vi "Initialize.vi"(8 "error in":errorcluster, 9 "Number of Channels":u32=1, 10 "Plugin Name":string, 11 "Voltage Limits in":refnum<class "Voltage Limits.lvclass">) -> (0 "error out":errorcluster, 3 "Voltage Limits out":refnum<class "Voltage Limits.lvclass">)   [LabVIEW 2023, in "Voltage Limits.lvclass"]
uses:
  Voltage Limits.lvclass
  Voltage Limits.lvclass/Voltage Limits.ctl
  <vilib>/ADAS Replay HIL/Channels/Tag Wrapper/Polymorphic/Open Consumer Tag (Double).vi
  <vilib>/ADAS Replay HIL/Channels/Tag Wrapper/Polymorphic/Set Default Value (Double).vi
  <vilib>/ADAS Replay HIL/Channels/Tag Wrapper/Polymorphic/Open Consumer Tag (Double).vi/bacb721e-673a-491a-accd-959f2e1f334e.vi
  <vilib>/ADAS Replay HIL/Channels/Tag Wrapper/Polymorphic/Set Default Value (Double).vi/228e99de-6fcf-414d-86fc-dc277c7b351f.vi
  <vilib>/ADAS Replay HIL/Channels/Tag Wrapper/Polymorphic/Open Consumer Tag (Double).vi/bacb721e-673a-491a-accd-959f2e1f334e.vi/c28b0ead-42ad-4072-80a2-aca7f2bd7ce3.vi
  <vilib>/ADAS Replay HIL/Channels/Tag Wrapper/Polymorphic/Set Default Value (Double).vi/228e99de-6fcf-414d-86fc-dc277c7b351f.vi/4bc1c15b-36ab-481f-b8dd-c64075ce723a.vi
  <vilib>/ADAS Replay HIL/AdasHilServices/AdasHilServices Fill In Error Info Ex.vi
  <vilib>/ADAS Replay HIL/Channels/Tag Wrapper/Tag Wrapper.lvlib
  Capability/Capability.lvclass
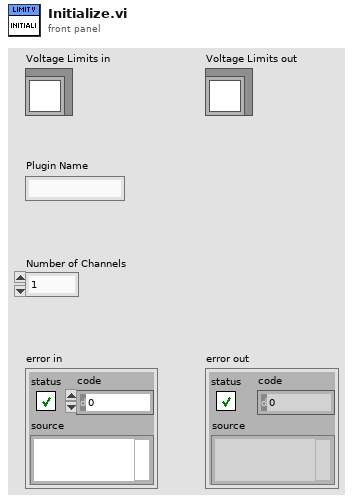
[diagram p1: front panel]
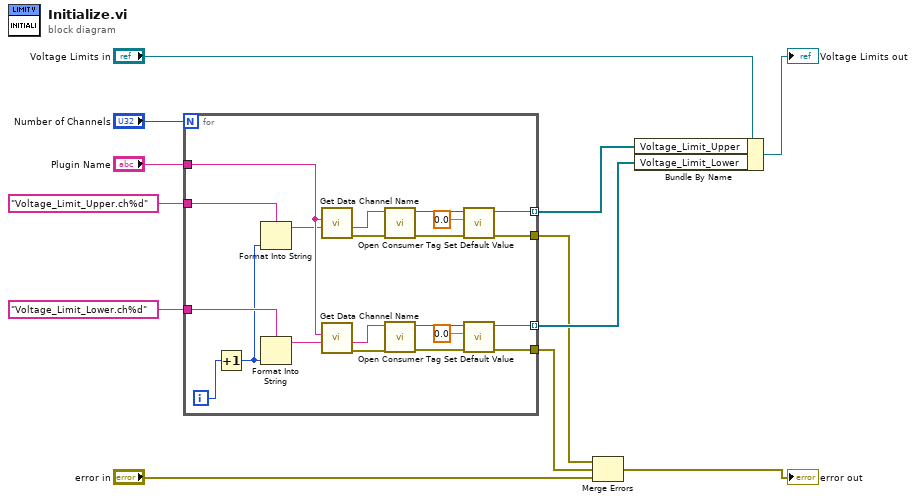
[diagram p0: block diagram]
diagram:
  n1 = for {
    N: "Number of Channels" -> [_]
    tunnel: [w29] -> w10 mode=indexing
    tunnel: [w28] -> w9 mode=indexing
    tunnel: [w27] -> w8
    tunnel: [w26] -> w7
    tunnel: "Plugin Name" -> [w25]
    tunnel: "Voltage_Limit_Upper.ch%d" ("Channel Name") -> [w17]
    tunnel: "Voltage_Limit_Lower.ch%d" ("Channel Name") -> [w15]
    i -> [w14]
    n2 = Increment(x=w14) -> (x+1=w13:i32)
    n3 = Format Into String(format string=w17, w13) -> (resulting string=w18:string)  [unwired: 2 in, 1 out]
    n4 = Format Into String(format string=w15, w13) -> (resulting string=w16:string)  [unwired: 2 in, 1 out]
    n5 = call "Get Data Channel Name.vi"("Channel Name"=w18, "Plugin Name"=w25) -> ("error out"=w22:errorcluster, "Data Channel Name"=w21:string)  [unwired: 8 in]
    n6 = call "Get Data Channel Name.vi"("Channel Name"=w16, "Plugin Name"=w25) -> ("error out"=w23:errorcluster, "Data Channel Name"=w24:string)  [unwired: 8 in]
    n7 = call-poly <vilib>:"Open Consumer Tag.vi"("error in"=w22, "Channel Name"=w21) -> ("error out"=w32:errorcluster, "ADAS HIL Channel"=w33:refnum<k21>)  [unwired: 8 in]
    n8 = call-poly <vilib>:"Open Consumer Tag.vi"("error in"=w23, "Channel Name"=w24) -> ("error out"=w30:errorcluster, "ADAS HIL Channel"=w31:refnum<k21>)  [unwired: 8 in]
    n9 = call-poly <vilib>:"Set Default Value.vi"("error in"=w32, "Default Value"=0.0, "ADAS HIL Channel in"=w33) -> ("error out"=w27:errorcluster, "ADAS HIL Channel out"=w29:refnum<k21>)  [unwired: 7 in]
    n10 = call-poly <vilib>:"Set Default Value.vi"("error in"=w30, "Default Value"=0.0, "ADAS HIL Channel in"=w31) -> ("error out"=w26:errorcluster, "ADAS HIL Channel out"=w28:refnum<k21>)  [unwired: 7 in]
  }
  n11 = Merge Errors(w8, w7, "error in") -> (→"error out":errorcluster)
  n12 = Bundle By Name(cluster="Voltage Limits in", "Voltage_Limit_Upper"=w10, "Voltage_Limit_Lower"=w9) -> (→"Voltage Limits out":refnum<class "Voltage Limits.lvclass">)
